vi "publishTel.vi"(8 "error in (no error)":errorcluster, 11 "TcpServer in":refnum<class "TcpServer.lvclass">) -> (0 "error out":errorcluster, 2 "telemetry flushed":string[](array[string]), 3 "TcpServer out":refnum<class "TcpServer.lvclass">)   [LabVIEW 2018]
doc: "Publish telemetry with a frecuency and a duration to TCP Client."
uses:
  TcpServer.lvclass
  TcpServer.lvclass/TcpServer.ctl
  TcpServerTel/TcpServerTel.lvclass/TcpServerTel.ctl
  TcpServerTel/TcpServerTel.lvclass
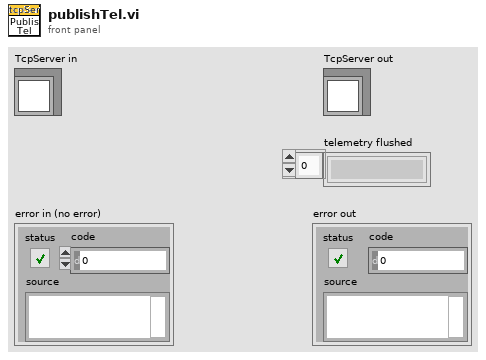
[diagram p1: front panel]
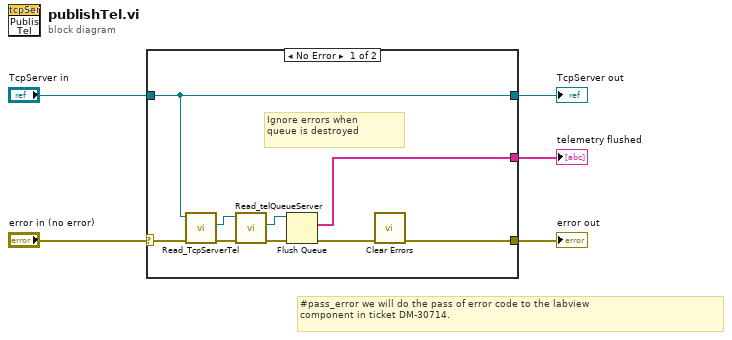
[diagram p0: block diagram]
diagram:
  # "#pass_error we will do the pass of error code to the labview \ncomponent in ticket DM-30714."
  n1 = case shown="No Error" "error in (no error)" {
    selector: "error in (no error)" -> [w9 w15]
    tunnel: [w14 _] -> w1
    tunnel: [w7 w15] -> w5
    tunnel: "TcpServer in" -> [w8 w16]
    tunnel: [w8 w16] -> w2
    frame No Error {
      # "Ignore errors when \nqueue is destroyed"
      n2 = call "Read_TcpServerTel.vi"("error in (no error)"=w9, "TcpServer in"=w8) -> ("error out"=w10:errorcluster, "TcpServerTel.lvclass"=w11:refnum<class "TcpServerTel.lvclass">)  [unwired: 7 in, 1 out]
      n3 = call "Read_telQueueServer.vi"("error in (no error)"=w10, "TcpServerTel in"=w11) -> ("error out"=w6:errorcluster, "telQueueServer"=w13:refnum<queue>)  [unwired: 7 in, 1 out]
      n4 = Flush Queue(queue=w13, error in (no error)=w6) -> (remaining elements=w14:string[], error out=w12:errorcluster)  [unwired: 1 out]
      n5 = call <vilib>:"Clear Errors.vi"("error in (no error)"=w12) -> ("error out"=w7:errorcluster)  [unwired: 5 in, 1 out]
    }
    frame Error {
    }
  }
  "error out" <- w5
  "TcpServer out" <- w2
  "telemetry flushed" <- w1
